vi "re_LuaVIEW Plug-in Handler.vi"(5 "LuaVIEW reference":T1, 11 "timeout (ms)":i32) -> (4 "handle":enum16{"timeout", "swap", "stop"}(ring))   [LabVIEW 2012]
doc: "This VI can be used inside a plug-in to assist in handling task signals. Examine the plugin template to see how it is deployed. The built-in handling of task signals does not work while called into a plug-in. Using this handler or similar code allows a plug-in to nevertheless respond to task signals. This handler limits itself to waiting for the timeout to expire when the plug-in was not started from a task."
uses:
  typedefs/t_LuaVIEW Reference.ctl
  typedefs/t_LuaVIEW Task State Methods.ctl
  typedefs/t_LuaVIEW Task Signals.ctl
  typedefs/t_LuaVIEW Task Modes.ctl
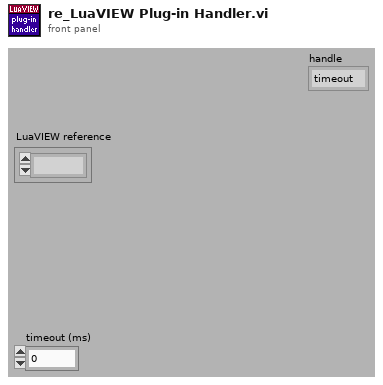
[diagram p1: front panel]
types:
  T1 = typedef "t_LuaVIEW Reference.ctl" = refnum<k1>
  T2 = typedef "t_LuaVIEW Task State Pane.ctl" = refnum<vi>
  T3 = typedef "t_LuaVIEW Task State Methods.ctl" = enum16{"cleanup", "set initial", "set mode", "set active mode", "set error", "get task info", "get script info", "set signal", "clear signal", "test handled", "test delegated", "test signal", "handle signal", "delegate signal", "allow signal", "disallow signal", "disallow all", "signals?", "delegated signals?", "protection++", "protection--", "protection=0", "message", "next message", "pop message", "message available?", "force stop", "set swap preps", "apply swap preps"}
  T4 = typedef "t_LuaVIEW Task Signals.ctl" = enum32{"resume", "pause", "swap", "stop", "confirm"}
  T5 = typedef "t_LuaVIEW Task Modes.ctl" = enum16{"initializing", "running", "executing", "paused", "error", "swapping"}
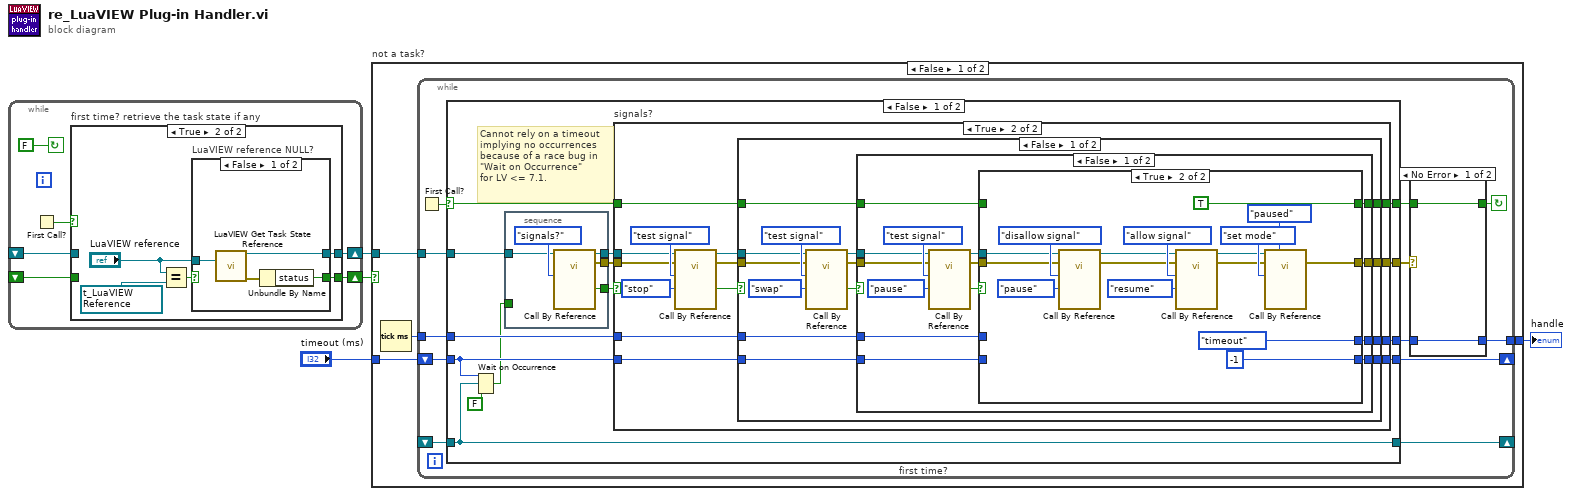
[diagram p0: block diagram]
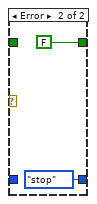
[diagram p4: hidden frame]
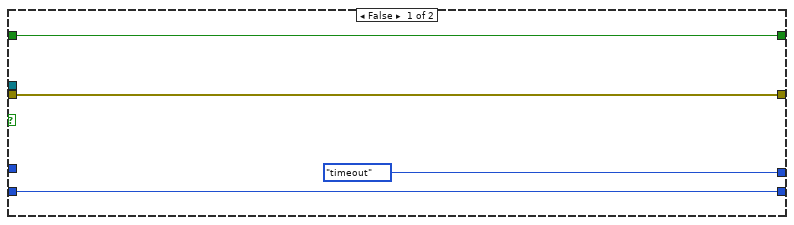
[diagram p5: hidden frame]
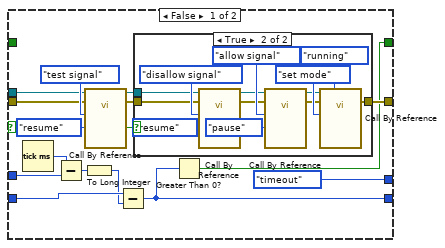
[diagram p6: hidden frame]
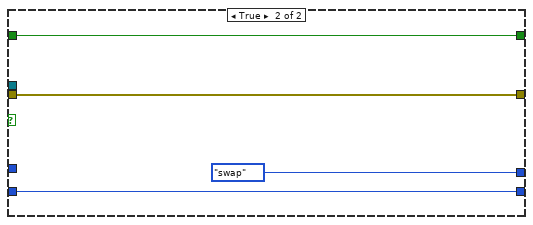
[diagram p8: hidden frame]
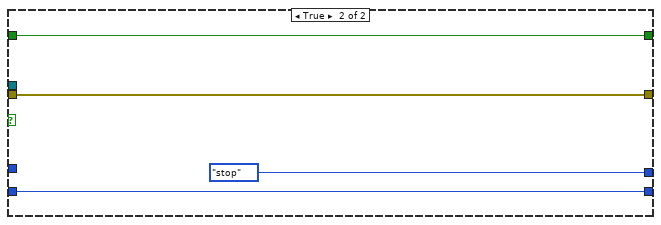
[diagram p9: hidden frame]
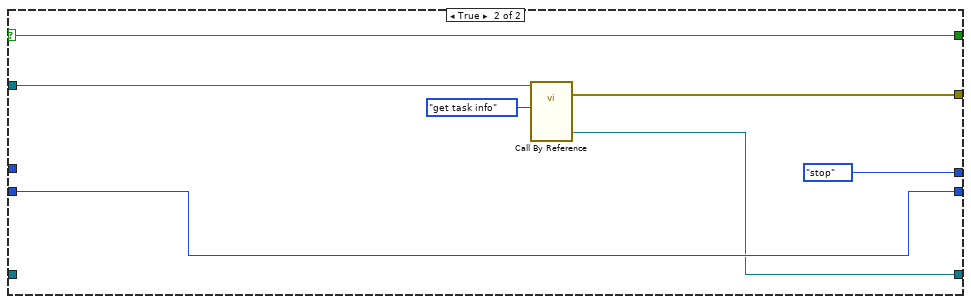
[diagram p10: hidden frame]
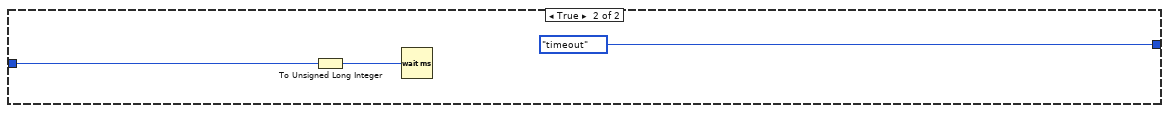
[diagram p11: hidden frame]
diagram:
  n1 = while {
    shift-right: [w10] -> w4
    shift-left: _ -> [w5]
    shift-right: [w9] -> w1
    shift-left: _ -> [w6]
    stop <- FALSE continue-if-true
    n2 = First Call?() -> (First Call?: T/F=w7:bool)
    n3 = case "first time? retrieve the task state if any" shown="True" w7 {
      tunnel: [w11 w17] -> w10
      tunnel: [w12 w16] -> w9
      tunnel: w6 -> [w12 _]
      tunnel: w5 -> [w11 _]
      frame False {
      }
      frame True {
        w15 = T1 refnum items=["LuaVIEW"] ("LuaVIEW reference")
        n4 = Equal?(x="LuaVIEW reference", y=w15) -> (x = y?=w13:bool)
        n5 = case "LuaVIEW reference NULL?" shown="False" w13 {
          selector: w13 -> [_ w22]
          tunnel: [w18 w22] -> w17
          tunnel: [w20 _] -> w16
          tunnel: "LuaVIEW reference" -> [w21 _]
          frame False {
            n6 = call "LuaVIEW Get Task State Reference.vi"("LuaVIEW reference in"=w21) -> ("task state reference"=w20:T2, "error out"=w19:errorcluster)  [unwired: 12 in, 1 out]
            n7 = Unbundle By Name(w19) -> ("status"=w18:bool)
          }
          frame True {
          }
        }
      }
    }
  }
  n8 = case "not a task?" shown="False" w4 {
    tunnel: w1 -> [w26 _]
    tunnel: "timeout (ms)" -> [w24 w170]
    tunnel: [w25 enum16{"timeout", "swap", "stop"}."timeout" ("handle")] -> w2
    frame False {
      n9 = Tick Count (ms)() -> (millisecond timer value=w23:u32)
      n10 = while {
        tunnel: w26 -> [w37]
        shift-right: [w27] -> _
        shift-left: _ -> [w36]
        tunnel: [w29] -> w25
        shift-right: [w34] -> _
        shift-left: w24 -> [w35]
        tunnel: w23 -> [w33]
        stop <- w30 continue-if-true
        n11 = First Call?() -> (First Call?: T/F=w38:bool)
        n12 = case "first time?" shown="False" w38 {
          selector: w38 -> [w55 w164]
          tunnel: w37 -> [w47 w168]
          tunnel: [w54 w164] -> w31
          tunnel: w36 -> [w49 _]
          tunnel: w35 -> [w48 w166]
          tunnel: [w53 enum16{"timeout", "swap", "stop"}."stop" ("handle")] -> w28
          tunnel: [w52 w166] -> w34
          tunnel: w33 -> [w51 _]
          tunnel: [w50 w165] -> w32
          tunnel: [w49 w163] -> w27
          frame False {
            # "Cannot rely on a timeout\nimplying no occurrences\nbecause of a race bug in\n\"Wait on Occurrence\"\nfor LV <= 7.1."
            n13 = Wait on Occurrence(1:FALSE ("ignore previous (T)"), 2:w49, 3:w48) -> (0:w43:bool)
            n14 = stacked-sequence {
              tunnel: w47 -> [w60]
              tunnel: [w59] -> w46
              tunnel: [w58] -> w45
              tunnel: [w57] -> w44
              tunnel: w43 -> [_]
              frame #0 {
                n15 = call-by-ref "?"(reference=w60, "method"=t_LuaVIEW_Task_State_Methods."signals?") -> (reference out=w58:T2, error out=w57:errorcluster, "set/available/pending"=w59:bool)  [unwired: 11 in, 4 out]
              }
            }
            n16 = case "signals?" shown="True" w46 {
              tunnel: w55 -> [w65 w78]
              tunnel: [w65 w77] -> w54
              tunnel: [enum16{"timeout", "swap", "stop"}."timeout" ("handle") w76] -> w53
              tunnel: [w63 w71] -> w52
              tunnel: w48 -> [w63 w73]
              tunnel: w51 -> [_ w72]
              tunnel: w45 -> [_ w67]
              tunnel: [w62 w70] -> w50
              tunnel: w44 -> [w62 w66]
              frame False {
              }
              frame True {
                n17 = call-by-ref "?"(reference=w67, error in=w66, "method"=t_LuaVIEW_Task_State_Methods."test signal", "signal"=t_LuaVIEW_Task_Signals."stop") -> (reference out=w75:T2, error out=w74:errorcluster, "set/available/pending"=w79:bool)  [unwired: 9 in, 4 out]
                n18 = case shown="False" w79 {
                  tunnel: w78 -> [w81 w161]
                  tunnel: [w82 w161] -> w77
                  tunnel: [w85 enum16{"timeout", "swap", "stop"}."stop" ("handle")] -> w76
                  tunnel: w75 -> [w91 _]
                  tunnel: w74 -> [w90 w158]
                  tunnel: w73 -> [w88 w159]
                  tunnel: w72 -> [w87 _]
                  tunnel: [w83 w159] -> w71
                  tunnel: [w80 w158] -> w70
                  frame False {
                    n19 = call-by-ref "?"(reference=w91, error in=w90, "method"=t_LuaVIEW_Task_State_Methods."test signal", "signal"=t_LuaVIEW_Task_Signals."swap") -> (reference out=w84:T2, error out=w86:errorcluster, "set/available/pending"=w89:bool)  [unwired: 9 in, 4 out]
                    n20 = case shown="False" w89 {
                      tunnel: w88 -> [w99 w155]
                      tunnel: w87 -> [w96 _]
                      tunnel: w86 -> [w105 w154]
                      tunnel: [w94 enum16{"timeout", "swap", "stop"}."swap" ("handle")] -> w85
                      tunnel: w84 -> [w104 _]
                      tunnel: [w102 w155] -> w83
                      tunnel: [w101 w156] -> w82
                      tunnel: w81 -> [w100 w156]
                      tunnel: [w95 w154] -> w80
                      frame False {
                        n21 = call-by-ref "?"(reference=w104, error in=w105, "method"=t_LuaVIEW_Task_State_Methods."test signal", "signal"=t_LuaVIEW_Task_Signals."pause") -> (reference out=w98:T2, error out=w97:errorcluster, "set/available/pending"=w103:bool)  [unwired: 9 in, 4 out]
                        n22 = case shown="True" w103 {
                          tunnel: [w108 -1 ("timeout (ms)")] -> w102
                          tunnel: [w109 TRUE] -> w101
                          tunnel: w100 -> [_ _]
                          tunnel: w99 -> [w113 _]
                          tunnel: w98 -> [w121 w142]
                          tunnel: w97 -> [w120 w139]
                          tunnel: w96 -> [w115 _]
                          tunnel: [w117 w147] -> w95
                          tunnel: [enum16{"timeout", "swap", "stop"}."timeout" ("handle") enum16{"timeout", "swap", "stop"}."timeout" ("handle")] -> w94
                          frame False {
                            n23 = Tick Count (ms)() -> (millisecond timer value=w114:u32)
                            n24 = Subtract(x=w114, y=w115) -> (x-y=w112:u32)
                            n25 = To Long Integer(number=w112) -> (32bit integer=w111:i32)
                            n26 = call-by-ref "?"(reference=w121, error in=w120, "method"=t_LuaVIEW_Task_State_Methods."test signal", "signal"=t_LuaVIEW_Task_Signals."resume") -> (reference out=w116:T2, error out=w118:errorcluster, "set/available/pending"=w119:bool)  [unwired: 9 in, 4 out]
                            n27 = Subtract(x=w113, y=w111) -> (x-y=w108:i32)
                            n28 = case shown="True" w119 {
                              tunnel: w118 -> [w124 w128]
                              tunnel: [w124 w132] -> w117
                              tunnel: w116 -> [_ w129]
                              frame False {
                              }
                              frame True {
                                n29 = call-by-ref "?"(reference=w129, error in=w128, "method"=t_LuaVIEW_Task_State_Methods."disallow signal", "signal"=t_LuaVIEW_Task_Signals."resume") -> (reference out=w127:T2, error out=w126:errorcluster)  [unwired: 9 in, 5 out]
                                n30 = call-by-ref "?"(reference=w127, error in=w126, "method"=t_LuaVIEW_Task_State_Methods."allow signal", "signal"=t_LuaVIEW_Task_Signals."pause") -> (reference out=w134:T2, error out=w133:errorcluster)  [unwired: 9 in, 5 out]
                                n31 = call-by-ref "?"(reference=w134, error in=w133, "method"=t_LuaVIEW_Task_State_Methods."set mode", "mode {set mode}"=t_LuaVIEW_Task_Modes."running" ("mode")) -> (error out=w132:errorcluster)  [unwired: 9 in, 6 out]
                              }
                            }
                            n32 = Greater Than 0?(x=w108) -> (x > 0?=w109:bool)
                          }
                          frame True {
                            n33 = call-by-ref "?"(reference=w142, error in=w139, "method"=t_LuaVIEW_Task_State_Methods."disallow signal", "signal"=t_LuaVIEW_Task_Signals."pause") -> (reference out=w141:T2, error out=w140:errorcluster)  [unwired: 9 in, 5 out]
                            n34 = call-by-ref "?"(reference=w141, error in=w140, "method"=t_LuaVIEW_Task_State_Methods."allow signal", "signal"=t_LuaVIEW_Task_Signals."resume") -> (reference out=w149:T2, error out=w148:errorcluster)  [unwired: 9 in, 5 out]
                            n35 = call-by-ref "?"(reference=w149, error in=w148, "method"=t_LuaVIEW_Task_State_Methods."set mode", "mode {set mode}"=t_LuaVIEW_Task_Modes."paused" ("mode")) -> (error out=w147:errorcluster)  [unwired: 9 in, 6 out]
                          }
                        }
                      }
                      frame True {
                      }
                    }
                  }
                  frame True {
                  }
                }
              }
            }
          }
          frame True {
            n36 = call-by-ref "?"(reference=w168, "method"=t_LuaVIEW_Task_State_Methods."get task info") -> (error out=w165:errorcluster, "wakeup occurrence"=w163:refnum<k4>)  [unwired: 11 in, 5 out]
          }
        }
        n37 = case shown="No Error" w32 {
          tunnel: w31 -> [w40 _]
          tunnel: [w40 FALSE] -> w30
          tunnel: [w39 enum16{"timeout", "swap", "stop"}."stop" ("handle")] -> w29
          tunnel: w28 -> [w39 _]
          frame No Error {
          }
          frame Error {
          }
        }
      }
    }
    frame True {
      n38 = To Unsigned Long Integer(number=w170) -> (unsigned 32bit integer=w169:u32)
      n39 = Wait (ms)(milliseconds to wait=w169) -> ()  [unwired: 1 out]
    }
  }
  "handle" <- w2
